vi "Control Center.vi"(7 "Center Style":T1(ring), 8 "Vertical":i32, 9 "Hor":i32, 10 "Control Re":refnum<vi>, 11 "PanelRef":refnum<vi>) -> (2 "Control Ref":refnum<vi>, 3 "Panel Ref":refnum<vi>)   [LabVIEW 2020]
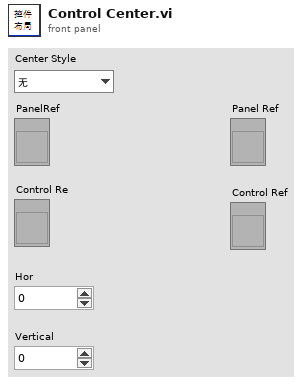
[diagram p1: front panel]
types:
  T1 = enum16{"无", "左边偏移", "右边偏移", "上偏移", "下偏移", "水平居中", "垂直居中", "水平&垂直居中", "匹配窗格"}
  T2 = typedef "LVBoundsTypeDef.ctl" = cluster{"Width":u32, "Height":u32}
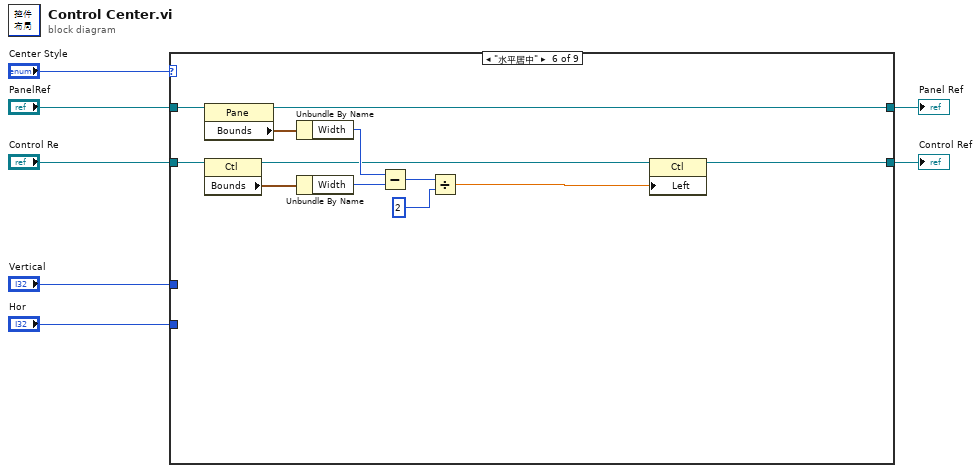
[diagram p0: block diagram]
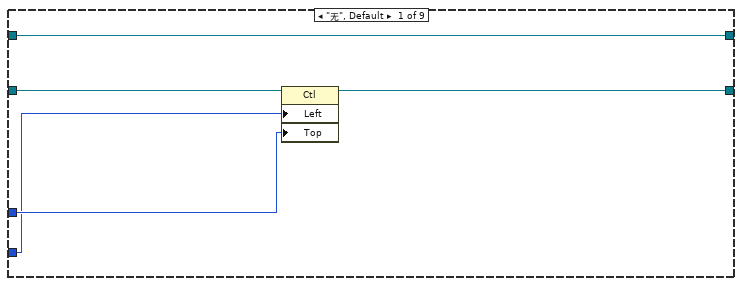
[diagram p2: hidden frame]
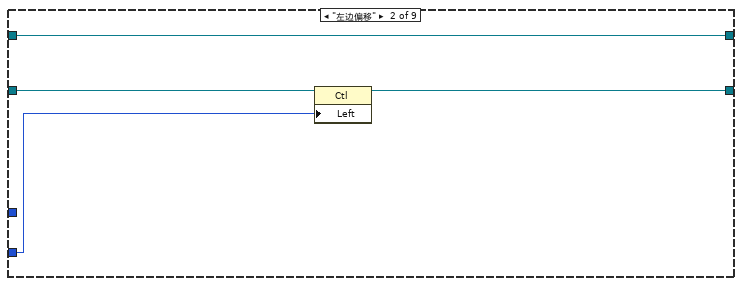
[diagram p3: hidden frame]
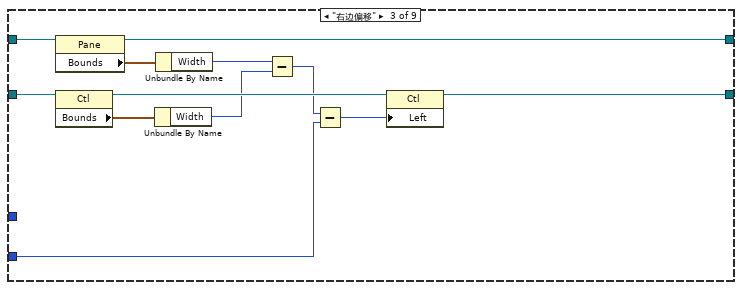
[diagram p4: hidden frame]
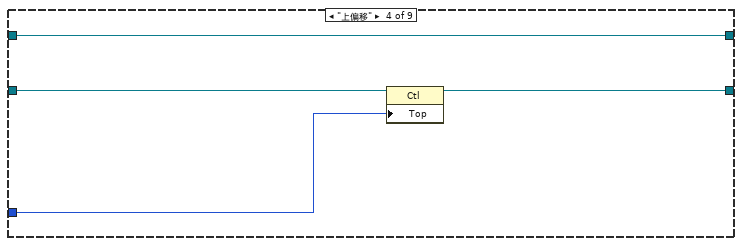
[diagram p5: hidden frame]
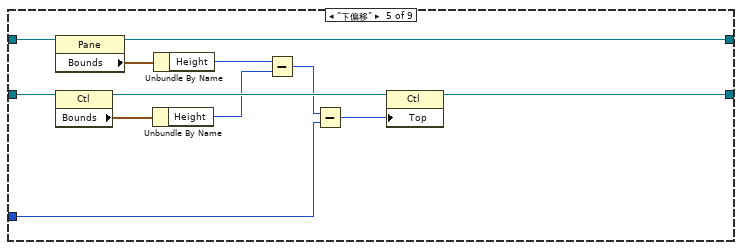
[diagram p6: hidden frame]
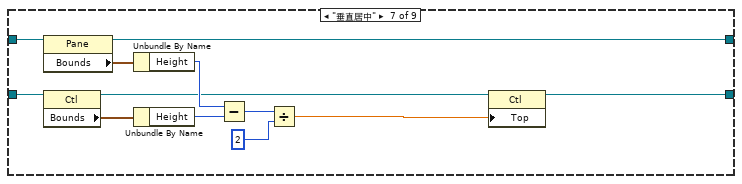
[diagram p7: hidden frame]
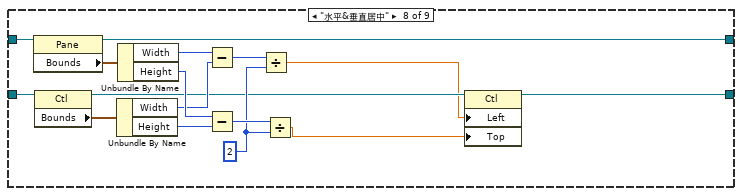
[diagram p8: hidden frame]
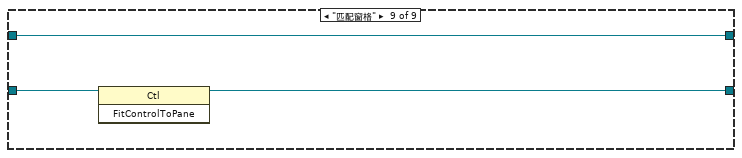
[diagram p9: hidden frame]
diagram:
  n1 = case shown="\"水平居中\"" "Center Style" {
    tunnel: "Control Re" -> [w11 w16 w23 w29 w39 w50 w62 w78 w87]
    tunnel: "Vertical" -> [w9 _ _ w31 w33 _ _ _ _]
    tunnel: "Hor" -> [w8 w13 w18 _ _ _ _ _ _]
    tunnel: "PanelRef" -> [w12 w14 w26 w30 w42 w52 w64 w79 w85]
    tunnel: [w12 w14 w25 w30 w41 w51 w63 w75 w85] -> w4
    tunnel: [w10 w15 w28 w32 w44 w47 w59 w71 w86] -> w3
    frame "无", Default {
      n2 = property class="Ctl"(reference=w11, "Left"=w8, "Top"=w9) -> (reference out=w10:refnum<vi>)  [unwired: 1 in, 1 out]
    }
    frame "左边偏移" {
      n3 = property class="Ctl"(reference=w16, "Left"=w13) -> (reference out=w15:refnum<vi>)  [unwired: 1 in, 1 out]
    }
    frame "右边偏移" {
      n4 = property class="Pane"(reference=w26) -> (reference out=w25:refnum<vi>, "Bounds"=w24:T2)  [unwired: 1 in, 1 out]
      n5 = property class="Ctl"(reference=w23) -> (reference out=w22:refnum<vi>, "Bounds"=w21:T2)  [unwired: 1 in, 1 out]
      n6 = Unbundle By Name(w21) -> ("Width"=w17:u32)
      n7 = Unbundle By Name(w24) -> ("Width"=w20:u32)
      n8 = Subtract(x=w20, y=w17) -> (x-y=w19:u32)
      n9 = Subtract(x=w19, y=w18) -> (x-y=w27:u32)
      n10 = property class="Ctl"(reference=w22, "Left"=w27) -> (reference out=w28:refnum<vi>)  [unwired: 1 in, 1 out]
    }
    frame "上偏移" {
      n11 = property class="Ctl"(reference=w29, "Top"=w31) -> (reference out=w32:refnum<vi>)  [unwired: 1 in, 1 out]
    }
    frame "下偏移" {
      n12 = property class="Pane"(reference=w42) -> (reference out=w41:refnum<vi>, "Bounds"=w40:T2)  [unwired: 1 in, 1 out]
      n13 = property class="Ctl"(reference=w39) -> (reference out=w38:refnum<vi>, "Bounds"=w37:T2)  [unwired: 1 in, 1 out]
      n14 = Unbundle By Name(w37) -> ("Height"=w34:u32)
      n15 = Unbundle By Name(w40) -> ("Height"=w36:u32)
      n16 = Subtract(x=w36, y=w34) -> (x-y=w35:u32)
      n17 = Subtract(x=w35, y=w33) -> (x-y=w43:u32)
      n18 = property class="Ctl"(reference=w38, "Top"=w43) -> (reference out=w44:refnum<vi>)  [unwired: 1 in, 1 out]
    }
    frame "水平居中" {
      n19 = property class="Pane"(reference=w52) -> (reference out=w51:refnum<vi>, "Bounds"=w46:T2)  [unwired: 1 in, 1 out]
      n20 = property class="Ctl"(reference=w50) -> (reference out=w48:refnum<vi>, "Bounds"=w49:T2)  [unwired: 1 in, 1 out]
      n21 = Unbundle By Name(w46) -> ("Width"=w56:u32)
      n22 = Unbundle By Name(w49) -> ("Width"=w55:u32)
      n23 = Subtract(x=w56, y=w55) -> (x-y=w54:u32)
      n24 = Divide(x=w54, y=u32 2) -> (x/y=w45:dbl)
      n25 = property class="Ctl"(reference=w48, "Left"=w45) -> (reference out=w47:refnum<vi>)  [unwired: 1 in, 1 out]
    }
    frame "垂直居中" {
      n26 = property class="Pane"(reference=w64) -> (reference out=w63:refnum<vi>, "Bounds"=w58:T2)  [unwired: 1 in, 1 out]
      n27 = property class="Ctl"(reference=w62) -> (reference out=w60:refnum<vi>, "Bounds"=w61:T2)  [unwired: 1 in, 1 out]
      n28 = Unbundle By Name(w58) -> ("Height"=w68:u32)
      n29 = Unbundle By Name(w61) -> ("Height"=w67:u32)
      n30 = Subtract(x=w68, y=w67) -> (x-y=w66:u32)
      n31 = Divide(x=w66, y=u32 2) -> (x/y=w57:dbl)
      n32 = property class="Ctl"(reference=w60, "Top"=w57) -> (reference out=w59:refnum<vi>)  [unwired: 1 in, 1 out]
    }
    frame "水平&垂直居中" {
      w80 = u32 2 ("y")
      n33 = property class="Pane"(reference=w79) -> (reference out=w75:refnum<vi>, "Bounds"=w77:T2)  [unwired: 1 in, 1 out]
      n34 = property class="Ctl"(reference=w78) -> (reference out=w72:refnum<vi>, "Bounds"=w76:T2)  [unwired: 1 in, 1 out]
      n35 = Unbundle By Name(w76) -> ("Width"=w74:u32, "Height"=w73:u32)
      n36 = Unbundle By Name(w77) -> ("Width"=w84:u32, "Height"=w82:u32)
      n37 = Subtract(x=w84, y=w74) -> (x-y=w83:u32)
      n38 = Subtract(x=w82, y=w73) -> (x-y=w81:u32)
      n39 = Divide(x=w83, y=w80) -> (x/y=w70:dbl)
      n40 = Divide(x=w81, y=w80) -> (x/y=w69:dbl)
      n41 = property class="Ctl"(reference=w72, "Left"=w70, "Top"=w69) -> (reference out=w71:refnum<vi>)  [unwired: 1 in, 1 out]
    }
    frame "匹配窗格" {
      n42 = invoke class="Ctl" method="FitControlToPane"(reference=w87) -> (reference out=w86:refnum<vi>)  [unwired: 2 in, 2 out]
    }
  }
  "Panel Ref" <- w4
  "Control Ref" <- w3
